vi "Table_SetTableFieldWidths.vi"(8 "error in (no error)":errorcluster, 10 "Widths":dbl[](array[numeric]), 11 "Listbox Ref":refnum<vi>) -> (0 "error out":errorcluster, 3 "Listbox Ref Out":refnum<vi>)   [LabVIEW 2012, in "TableSupportLib.lvlib"]
uses:
  TableSupportLib.lvlib
  <vilib>/Utility/miscctls.llb/LVRowAndColumnTypeDef.ctl
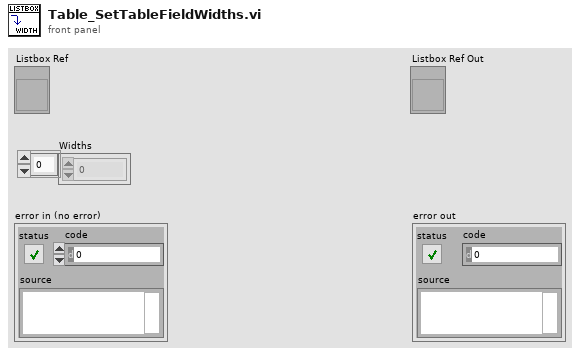
[diagram p1: front panel]
types:
  T1 = typedef "LVRowAndColumnTypeDef.ctl" = cluster{"Row":i32, "Column":i32}
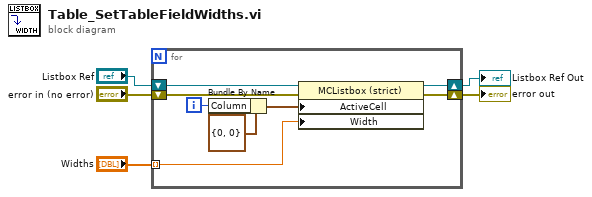
[diagram p0: block diagram]
diagram:
  n1 = for {
    tunnel: "Widths" -> [w13] mode=indexing
    shift-right: [w7] -> w5
    shift-left: "error in (no error)" -> [w8]
    shift-right: [w6] -> w1
    shift-left: "Listbox Ref" -> [w9]
    i -> [w10]
    n2 = Bundle By Name(cluster=T1 {"Row"=0, "Column"=0} ("Active Cell:Active Cell"), "Column"=w10) -> (w11:T1)
    n3 = property on="Property Node" class="MCListbox (strict)"(reference=w9, error in=w8, "ActiveCell"=w11, "Width"=w13) -> (reference out=w6:refnum<vi>, error out=w7:errorcluster)
  }
  "error out" <- w5
  "Listbox Ref Out" <- w1
